vi "Find Subpanel on Page.vi"(8 "error in (no error)":errorcluster, 11 "Page in":refnum<vi>) -> (0 "error out":errorcluster, 2 "Sub panel reference":refnum<vi>, 3 "Page out":refnum<vi>)   [LabVIEW 2020]
panel:
  in  "Sub Panel":refnum<vi>
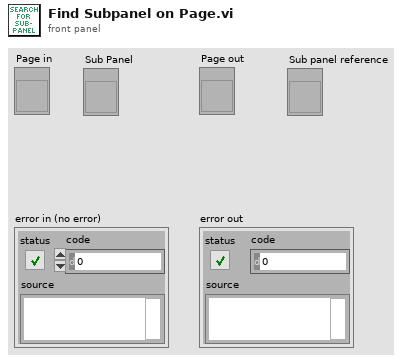
[diagram p1: front panel]
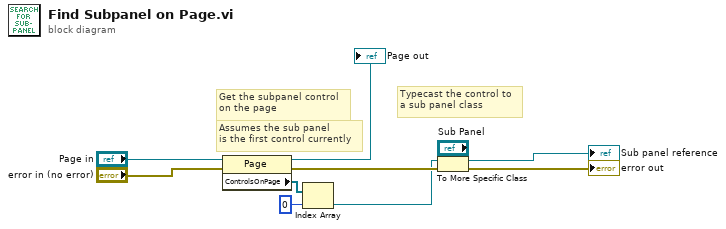
[diagram p0: block diagram]
diagram:
  # "Typecast the control to\na sub panel class"
  # "Assumes the sub panel\nis the first control currently"
  # "Get the subpanel control\non the page"
  n1 = property class="Page"(reference="Page in", error in="error in (no error)") -> (reference out=→"Page out":refnum<vi>, error out=w4:errorcluster, "ControlsOnPage"=w9:refnum<vi>[])
  n2 = Index Array(array=w9, index=0) -> (element=w3:refnum<vi>)
  n3 = To More Specific Class(target class="Sub Panel", reference=w3, error in=w4) -> (specific class reference=→"Sub panel reference":refnum<vi>, error out=→"error out":errorcluster)
